vi "Set Point Sliders.vi"() -> ()   [LabVIEW 2013]
panel:
  in  "Z Position Set Point":dbl(slide) min=0.0 max=15000.0 scale=0.0..10.0
  in  "Y Position Set Point":dbl(slide) min=0.0 max=15000.0 scale=0.0..10.0
  in  "X Position Set Point":dbl(slide) min=0.0 max=15000.0 scale=0.0..10.0
  # "X"
  # "Y"
  # "Z"
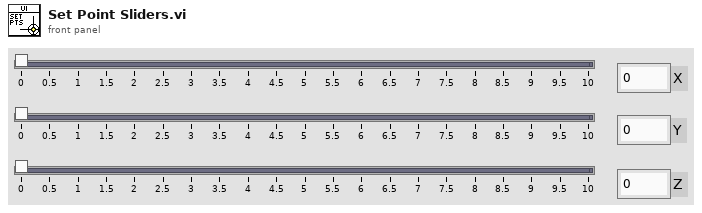
[diagram p1: front panel]
types:
  T1 = enum8{"Enabled", "Disabled", "Disabled and Grayed Out"}
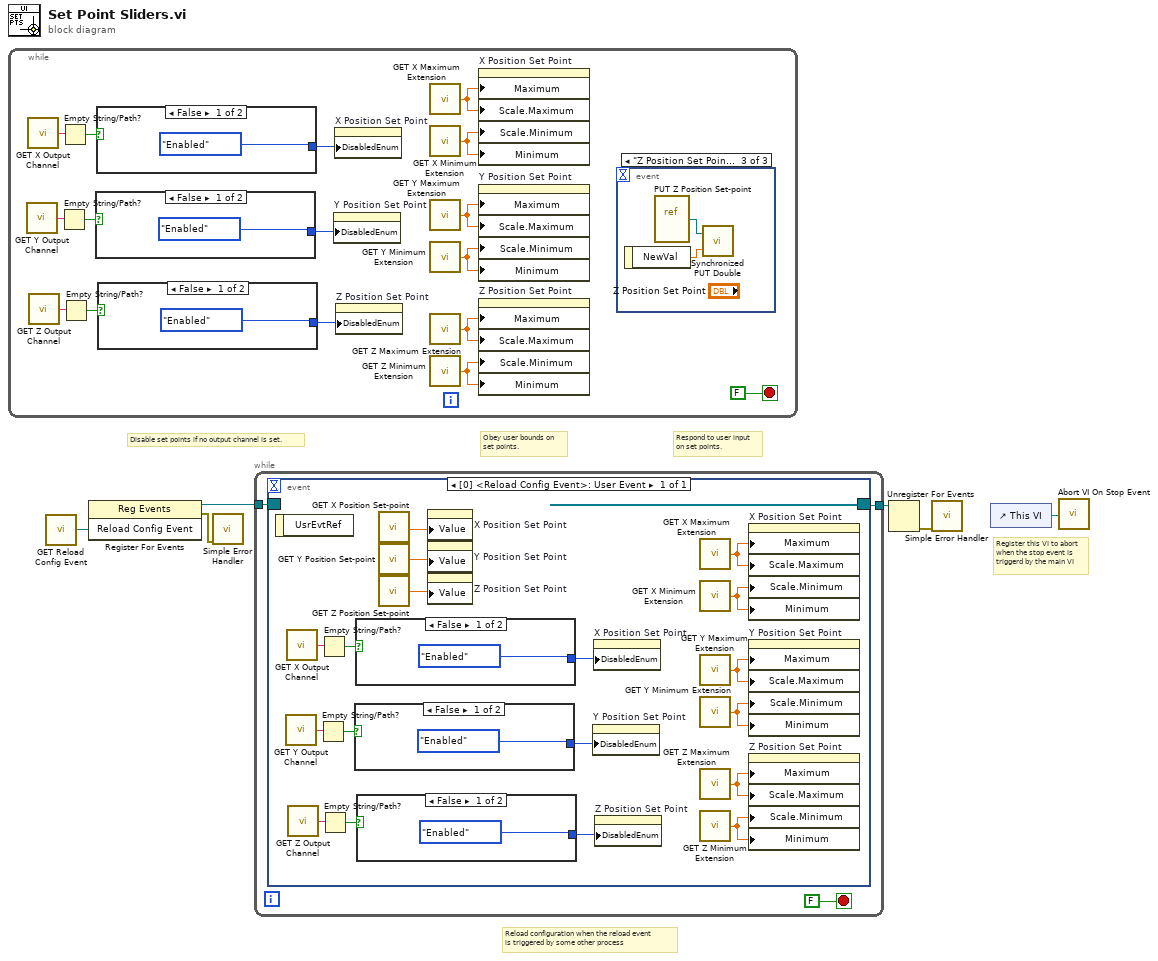
[diagram p0: block diagram]
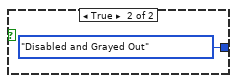
[diagram p2: hidden frame]
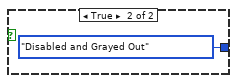
[diagram p3: hidden frame]
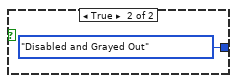
[diagram p4: hidden frame]
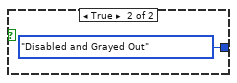
[diagram p5: hidden frame]
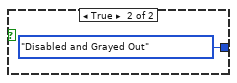
[diagram p6: hidden frame]
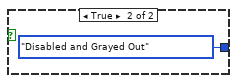
[diagram p7: hidden frame]
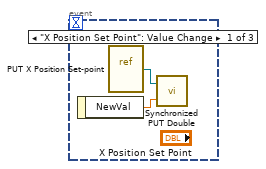
[diagram p8: hidden frame]
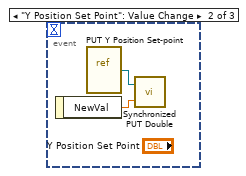
[diagram p9: hidden frame]
diagram:
  # "Reload configuration when the reload event\nis triggered by some other process"
  # "Register this VI to abort\nwhen the stop event is\ntriggerd by the main VI"
  # "Disable set points if no output channel is set."
  # "Respond to user input\non set points."
  # "Obey user bounds on\nset points."
  n1 = while {
    stop <- FALSE stop-if-true
    n2 = call "GET Y Output Channel.vi"() -> ("Y Output Channel"=w18:string)
    n3 = call "GET X Output Channel.vi"() -> ("X Output Channel"=w21:string)
    n4 = call "GET Z Output Channel.vi"() -> ("Z Output Channel"=w15:string)
    n5 = Empty String/Path?(string/path=w18) -> (empty?=w17:bool)
    n6 = Empty String/Path?(string/path=w21) -> (empty?=w20:bool)
    n7 = Empty String/Path?(string/path=w15) -> (empty?=w14:bool)
    n8 = case shown="False" w17 {
      tunnel: [T1."Enabled" ("Disabled") T1."Disabled and Grayed Out" ("Disabled")] -> w16
      frame False {
      }
      frame True {
      }
    }
    n9 = case shown="False" w20 {
      tunnel: [T1."Enabled" ("Disabled") T1."Disabled and Grayed Out" ("Disabled")] -> w19
      frame False {
      }
      frame True {
      }
    }
    n10 = case shown="False" w14 {
      tunnel: [T1."Enabled" ("Disabled") T1."Disabled and Grayed Out" ("Disabled")] -> w13
      frame False {
      }
      frame True {
      }
    }
    n11 = property on="Y Position Set Point" class="Slide (strict)"("DisabledEnum"=w16) -> ()  [unwired: 2 in, 2 out]
    n12 = property on="X Position Set Point" class="Slide (strict)"("DisabledEnum"=w19) -> ()  [unwired: 2 in, 2 out]
    n13 = property on="Z Position Set Point" class="Slide (strict)"("DisabledEnum"=w13) -> ()  [unwired: 2 in, 2 out]
    n14 = call "GET X Maximum Extension.vi"() -> ("X Maximum Extension"=w7:dbl)
    n15 = call "GET X Minimum Extension.vi"() -> ("X Minimum Extension"=w8:dbl)
    n16 = call "GET Y Maximum Extension.vi"() -> ("Y Maximum Extension"=w10:dbl)
    n17 = call "GET Y Minimum Extension.vi"() -> ("Y Minimum Extension"=w9:dbl)
    n18 = call "GET Z Maximum Extension.vi"() -> ("Z Maximum Extension"=w11:dbl)
    n19 = call "GET Z Minimum Extension.vi"() -> ("Z Minimum Extension"=w12:dbl)
    n20 = property on="X Position Set Point" class="Slide (strict)"("Maximum"=w7, "Scale.Maximum"=w7, "Scale.Minimum"=w8, "Minimum"=w8) -> ()  [unwired: 2 in, 2 out]
    n21 = property on="Y Position Set Point" class="Slide (strict)"("Maximum"=w10, "Scale.Maximum"=w10, "Scale.Minimum"=w9, "Minimum"=w9) -> ()  [unwired: 2 in, 2 out]
    n22 = property on="Z Position Set Point" class="Slide (strict)"("Maximum"=w11, "Scale.Maximum"=w11, "Scale.Minimum"=w12, "Minimum"=w12) -> ()  [unwired: 2 in, 2 out]
    n23 = event shown="[2] \"Z Position Set Point\": Value Change" {
      selector: _ -> [_ _ _]
      dyn-events: _ -> [_ _ _]
      timeout: _ -> [_ _ _]
      event "X Position Set Point": Value Change {
        n24 = event-data() -> ("NewVal"=w29:dbl)  [unwired: 1 in]
        n25 = vi-ref "PUT X Position Set-point.vi"() -> (w30:refnum<vi>)
        n26 = call "Synchronized PUT Double.vi"("PUT Value"=w29, "PUT VI Reference"=w30) -> ()  [unwired: 1 in]
      }
      event "Y Position Set Point": Value Change {
        n27 = event-data() -> ("NewVal"=w31:dbl)  [unwired: 1 in]
        n28 = vi-ref "PUT Y Position Set-point.vi"() -> (w32:refnum<vi>)
        n29 = call "Synchronized PUT Double.vi"("PUT Value"=w31, "PUT VI Reference"=w32) -> ()  [unwired: 1 in]
      }
      event "Z Position Set Point": Value Change {
        n30 = event-data() -> ("NewVal"=w33:dbl)  [unwired: 1 in]
        n31 = vi-ref "PUT Z Position Set-point.vi"() -> (w34:refnum<vi>)
        n32 = call "Synchronized PUT Double.vi"("PUT Value"=w33, "PUT VI Reference"=w34) -> ()  [unwired: 1 in]
      }
    }
  }
  n33 = call "GET Reload Config Event.vi"() -> ("Reload Config Event"=w5:refnum<user-event>)
  n34 = register-events(w5) -> (reference out=w4:refnum<event-registration>, error out=w3:errorcluster)  [unwired: 2 in]
  n35 = call <vilib>:"Simple Error Handler.vi"("error in (no error)"=w3) -> ()  [unwired: 4 in, 5 out]
  n36 = while {
    tunnel: [w37] -> w2
    tunnel: w4 -> [w36]
    stop <- FALSE stop-if-true
    n37 = event shown="[0] <Reload Config Event>: User Event" {
      selector: w36 -> [_]
      dyn-events: [_] -> w37
      timeout: _ -> [_]
      event User Event {
        n38 = event-data() -> ()  [unwired: 1 in, 1 out]
        n39 = call "GET Y Output Channel.vi"() -> ("Y Output Channel"=w47:string)
        n40 = call "GET X Output Channel.vi"() -> ("X Output Channel"=w44:string)
        n41 = call "GET Z Output Channel.vi"() -> ("Z Output Channel"=w50:string)
        n42 = Empty String/Path?(string/path=w47) -> (empty?=w48:bool)
        n43 = Empty String/Path?(string/path=w44) -> (empty?=w45:bool)
        n44 = Empty String/Path?(string/path=w50) -> (empty?=w51:bool)
        n45 = case shown="False" w48 {
          tunnel: [T1."Enabled" ("Disabled") T1."Disabled and Grayed Out" ("Disabled")] -> w49
          frame False {
          }
          frame True {
          }
        }
        n46 = case shown="False" w45 {
          tunnel: [T1."Enabled" ("Disabled") T1."Disabled and Grayed Out" ("Disabled")] -> w46
          frame False {
          }
          frame True {
          }
        }
        n47 = case shown="False" w51 {
          tunnel: [T1."Enabled" ("Disabled") T1."Disabled and Grayed Out" ("Disabled")] -> w52
          frame False {
          }
          frame True {
          }
        }
        n48 = call "GET X Position Set-point.vi"() -> ("X Position Set-point"=w55:dbl)
        n49 = call "GET Y Position Set-point.vi"() -> ("Y Position Set-point"=w54:dbl)
        n50 = call "GET Z Position Set-point.vi"() -> ("Z Position Set-point"=w53:dbl)
        n51 = property on="X Position Set Point" class="Slide (strict)"("Value"=w55) -> ()  [unwired: 2 in, 2 out]
        n52 = property on="Y Position Set Point" class="Slide (strict)"("Value"=w54) -> ()  [unwired: 2 in, 2 out]
        n53 = property on="Z Position Set Point" class="Slide (strict)"("Value"=w53) -> ()  [unwired: 2 in, 2 out]
        n54 = property on="Y Position Set Point" class="Slide (strict)"("DisabledEnum"=w49) -> ()  [unwired: 2 in, 2 out]
        n55 = property on="X Position Set Point" class="Slide (strict)"("DisabledEnum"=w46) -> ()  [unwired: 2 in, 2 out]
        n56 = property on="Z Position Set Point" class="Slide (strict)"("DisabledEnum"=w52) -> ()  [unwired: 2 in, 2 out]
        n57 = call "GET X Maximum Extension.vi"() -> ("X Maximum Extension"=w43:dbl)
        n58 = call "GET X Minimum Extension.vi"() -> ("X Minimum Extension"=w42:dbl)
        n59 = call "GET Y Maximum Extension.vi"() -> ("Y Maximum Extension"=w40:dbl)
        n60 = call "GET Y Minimum Extension.vi"() -> ("Y Minimum Extension"=w41:dbl)
        n61 = call "GET Z Maximum Extension.vi"() -> ("Z Maximum Extension"=w39:dbl)
        n62 = call "GET Z Minimum Extension.vi"() -> ("Z Minimum Extension"=w38:dbl)
        n63 = property on="X Position Set Point" class="Slide (strict)"("Maximum"=w43, "Scale.Maximum"=w43, "Scale.Minimum"=w42, "Minimum"=w42) -> ()  [unwired: 2 in, 2 out]
        n64 = property on="Y Position Set Point" class="Slide (strict)"("Maximum"=w40, "Scale.Maximum"=w40, "Scale.Minimum"=w41, "Minimum"=w41) -> ()  [unwired: 2 in, 2 out]
        n65 = property on="Z Position Set Point" class="Slide (strict)"("Maximum"=w39, "Scale.Maximum"=w39, "Scale.Minimum"=w38, "Minimum"=w38) -> ()  [unwired: 2 in, 2 out]
      }
    }
  }
  n66 = Unregister For Events(event registration refnum=w2) -> (error out=w1:errorcluster)  [unwired: 1 in]
  n67 = call <vilib>:"Simple Error Handler.vi"("error in (no error)"=w1) -> ()  [unwired: 4 in, 5 out]
  n68 = control-ref of="This VI"() -> (w6:refnum<vi>)
  n69 = call "Abort VI On Stop Event.vi"("VI Reference"=w6) -> ()
